vi "Buffer Initialize.vi"(8 "error in (no error)":errorcluster, 9 "Number Of Elements":i32[](array[numeric]), 10 "Sector Number":i32, 11 "Circular Buffer 1D U16 DVR Queue in":refnum<class "Circular Buffer 1D U16 DVR Queue.lvclass">) -> (0 "error out":errorcluster, 3 "Circular Buffer 1D U16 DVR Queue out":refnum<class "Circular Buffer 1D U16 DVR Queue.lvclass">)   [LabVIEW 2024, in "Circular Buffer 1D U16 DVR Queue.lvclass"]
uses:
  Circular Buffer 1D U16 DVR Queue.lvclass
  Type Def/1D U16 DVR.ctl
  Circular Buffer 1D U16 DVR Queue.lvclass/Circular Buffer 1D U16 DVR Queue.ctl
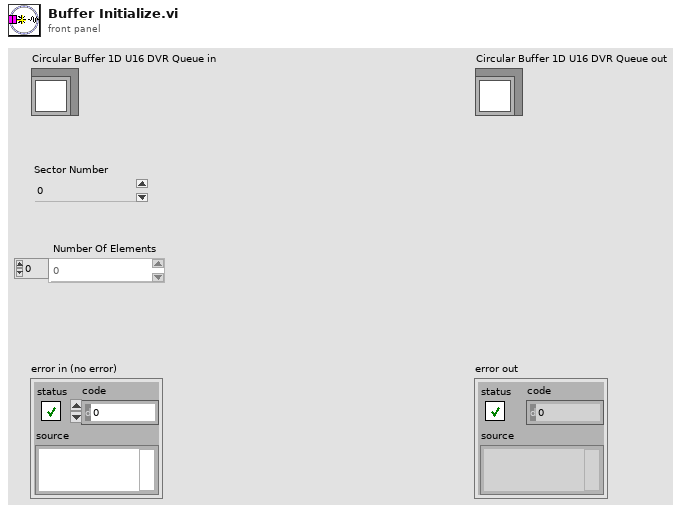
[diagram p1: front panel]
types:
  T1 = typedef "1D U16 DVR.ctl" = refnum<data-value>
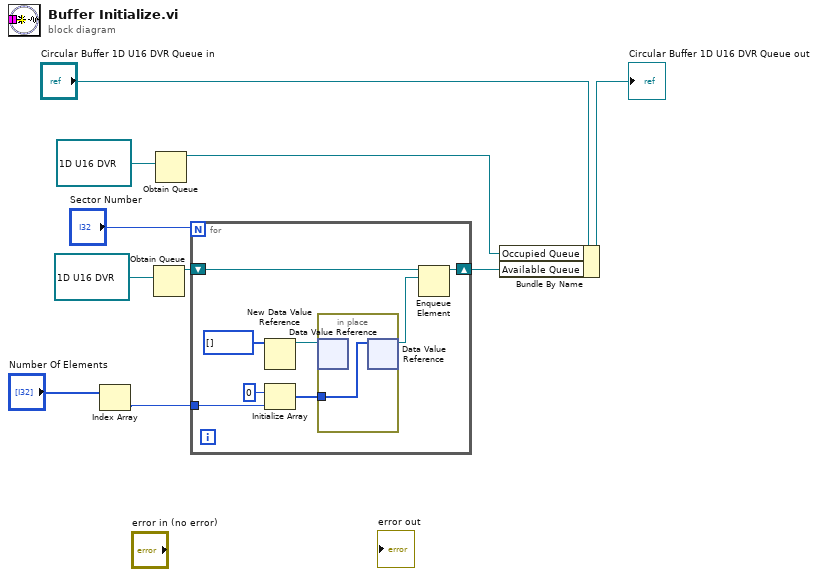
[diagram p0: block diagram]
diagram:
  n1 = Index Array(array="Number Of Elements") -> (element=w1:i32)  [unwired: 1 in]
  n2 = Obtain Queue(element data type=T1 refnum ("1D U16 DVR")) -> (queue out=w8:refnum<queue>)  [unwired: 4 in, 2 out]
  n3 = Obtain Queue(element data type=T1 refnum ("1D U16 DVR")) -> (queue out=w4:refnum<queue>)  [unwired: 4 in, 2 out]
  n4 = for {
    N: "Sector Number" -> [_]
    tunnel: w1 -> [w17]
    shift-right: [w11] -> w5
    shift-left: w8 -> [w13]
    n5 = New Data Value Reference(data value=u16[] [] ("initialized array")) -> (data value reference=w15:refnum<data-value>)  [unwired: 1 in, 1 out]
    n6 = Initialize Array(u16 0 ("element"), w17) -> (w14:u16[])
    n7 = in-place {
      in-place-border: w14 -> [w19]
      n8 = in-place-dvr #1(w15) -> ()  [unwired: 2 out]
      n9 = in-place-dvr #1(w19) -> (w12:refnum<data-value>)  [unwired: 1 out]
    }
    n10 = Enqueue Element(queue=w13, element=w12) -> (queue out=w11:refnum<queue>)  [unwired: 2 in, 2 out]
  }
  n11 = Bundle By Name(cluster="Circular Buffer 1D U16 DVR Queue in", "Occupied Queue"=w4, "Available Queue"=w5) -> (→"Circular Buffer 1D U16 DVR Queue out":refnum<class "Circular Buffer 1D U16 DVR Queue.lvclass">)
